vi "Sonic Systems P100 Test Program.vi"() -> ()   [LabVIEW 2018, in "Sonic Systems P100.lvlib"]
uses:
  Sonic Systems P100.lvlib
  Sonic Systems P100 Settings.ctl
panel:
  out "Running":bool
  out "Connection Error":bool
  in  "stop":bool
  in  "Amplitude":dbl
  in  "Run":bool
  out "error out":errorcluster
  in  "error in (no error)":errorcluster
  out "SS P100 Settings":T1
  in  "SS P100 Settings":T1
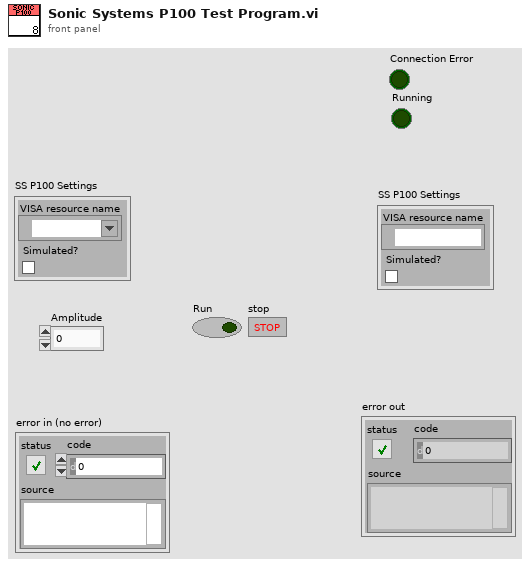
[diagram p1: front panel]
types:
  T1 = typedef "Sonic Systems P100.lvlib/Sonic Systems P100 Settings.ctl" = cluster{"VISA resource name":refnum<visa-resource-name>, "Simulated?":bool}
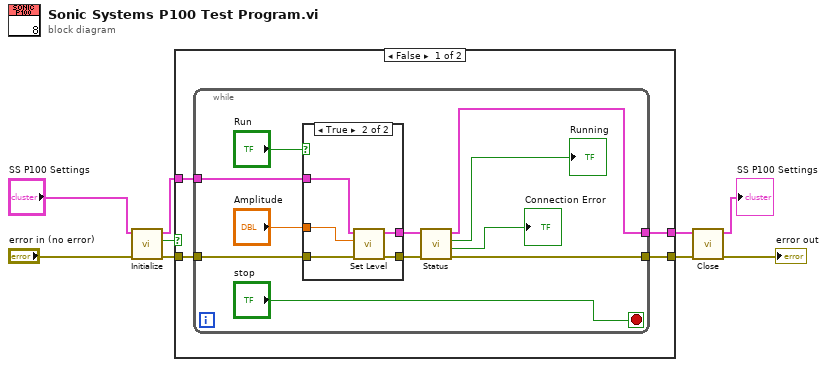
[diagram p0: block diagram]
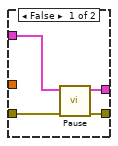
[diagram p2: hidden frame]
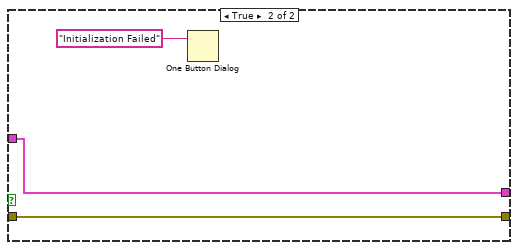
[diagram p3: hidden frame]
diagram:
  n1 = call "Initialize.vi"("error in (no error)"="error in (no error)", "SS P100 Settings"="SS P100 Settings") -> ("error out"=w2:errorcluster, "Connection Error"=w1:bool, "SS P100 Settings"=w3:T1)  [unwired: 7 in]
  n2 = case shown="False" w1 {
    tunnel: [w13 w35] -> w7
    tunnel: [w12 w34] -> w5
    tunnel: w3 -> [w11 w35]
    tunnel: w2 -> [w10 w34]
    frame False {
      n3 = while {
        tunnel: [w24] -> w13
        tunnel: [w23] -> w12
        tunnel: w11 -> [w21]
        tunnel: w10 -> [w20]
        stop <- "stop" stop-if-true
        n4 = case shown="True" "Run" {
          tunnel: w21 -> [w28 w33]
          tunnel: w20 -> [w27 w32]
          tunnel: [w26 w31] -> w19
          tunnel: [w25 w30] -> w18
          tunnel: "Amplitude" -> [_ w29]
          frame False {
            n5 = call "Pause.vi"("error in (no error)"=w27, "SS P100 Settings In"=w28) -> ("error out"=w26:errorcluster, "SS P100 Settings Out"=w25:T1)  [unwired: 8 in]
          }
          frame True {
            n6 = call "Set Level.vi"("error in (no error)"=w32, "Setpoint"=w29, "SS P100 Settings In"=w33) -> ("error out"=w31:errorcluster, "SS P100 Settings Out"=w30:T1)  [unwired: 6 in, 1 out]
          }
        }
        n7 = call "Status.vi"("error in (no error)"=w19, "SS P100 Settings In"=w18) -> ("error out"=w23:errorcluster, "Connection Error"=→"Connection Error":bool, "Running"=→"Running":bool, "SS P100 Settings Out"=w24:T1)  [unwired: 4 in, 2 out]
      }
    }
    frame True {
      n8 = One Button Dialog(message="Initialization Failed") -> ()  [unwired: 1 in, 1 out]
    }
  }
  n9 = call "Close.vi"("error in (no error)"=w5, "SS P100 Settings"=w7) -> ("error out"=→"error out":errorcluster, "SS P100 Settings"=→"SS P100 Settings":T1)  [unwired: 8 in]
